vi "PID FRC form.vi"(4 "reinitialize? (F)":bool, 5 "output range":cluster{"output high":dbl, "output low":dbl}={"output high"=1.0, "output low"=-1.0} {"output low" format="%.2f"; "output high" format="%.2f"}, 6 "dt (s)":dbl=-1.0 format="%.3f", 7 "setpoint":dbl format="%.2f", 8 "d smoothing":dbl=nan format="%.2f", 9 "Feed Forward":dbl=1.5000000000000002, 10 "process variable":dbl format="%.2f", 11 "PID gains":T1={"proportional (Kc)"=1.0, "integral (Ki)"=0.01, "derivative (Kd)"=0.0} {"derivative (Kd)" format="%.3f"; "integral (Ki)" format="%.3f"; "proportional (Kc)" format="%.3f"}) -> (0 "dt out (s)":dbl format="%.3f", 1 "Chart":cluster{dbl, dbl}(graph), 3 "output":dbl format="%.2f")   [LabVIEW 2020]
doc: "Implements a PID that better meets FRC needs. It is in parallel form (Kp, Ki, Kd) and includes an arbitrary feedforward that is added to the output.\nThe PID algorithm features control output range limiting with integrator anti-windup and bumpless controller output for PID gain changes. The d smoothing (0-1) can help avoid oscillations caused by a stronger d term."
uses:
  <vilib>/addons/control/pid/pid.llb/PID Structure.ctl
  <vilib>/addons/control/pid/pid.llb/PID Structure Conversion (DBL).vi
  <vilib>/addons/control/pid/pid.llb/PID Advanced (DBL).vi
  <vilib>/addons/control/pid/NI_PID_pid.lvlib
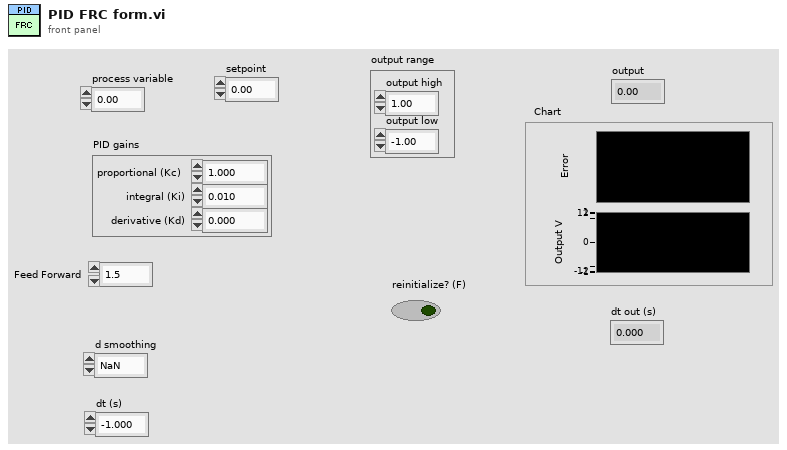
[diagram p1: front panel]
types:
  T1 = cluster{"proportional (Kc)":dbl, "integral (Ki)":dbl, "derivative (Kd)":dbl}
  T2 = typedef "NI_PID_pid.lvlib/PID Structure.ctl" = u16
  T3 = cluster{"proportional gain (Kc)":dbl, "integral time (Ti, min)":dbl, "derivative time (Td, min)":dbl}
  T4 = cluster{"proportional gain (Kc)":bool, "integral time (Ti, min)":bool, "derivative time (Td, min)":bool}
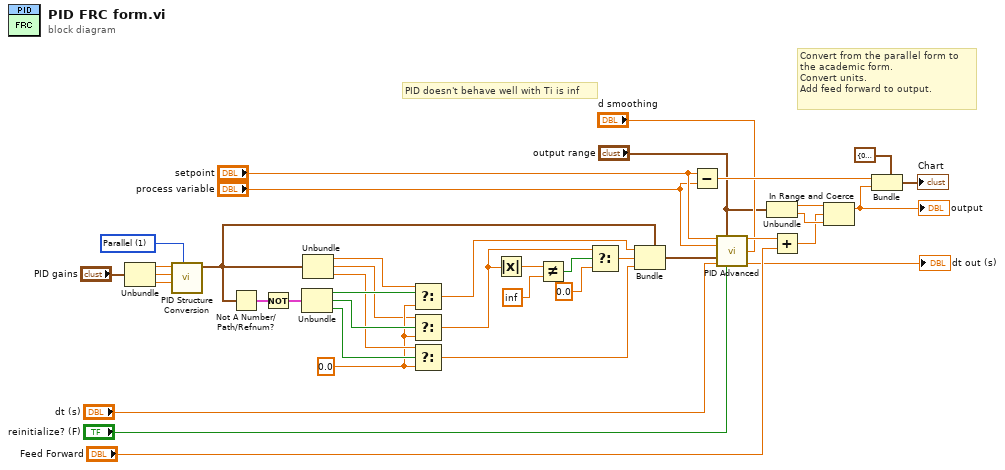
[diagram p0: block diagram]
diagram:
  w23 = 0.0
  w40 = T2 1 items=["Academic (Standard)", "Parallel", "Series"] ("PID structure")
  # "PID doesn't behave well with Ti is inf"
  # "Convert from the parallel form to\nthe academic form.\nConvert units.\nAdd feed forward to output."
  n1 = Unbundle("PID gains") -> ("proportional (Kc)"=w38:dbl, "integral (Ki)"=w37:dbl, "derivative (Kd)"=w36:dbl)
  n2 = call-poly <vilib>:"PID Structure Conversion.vi"("PID structure"=w40, "derivative"=w36, "integral"=w37, "proportional"=w38) -> ("PID gains"=w31:T3)  [unwired: 7 in]
  n3 = Not A Number/Path/Refnum?(number/path/refnum=w31) -> (NaN/Path/Refnum?=w30:T4)
  n4 = Not(x=w30) -> (.not. x?=w28:T4)
  n5 = Unbundle(w28) -> ("proportional gain (Kc)"=w29:bool, "integral time (Ti, min)"=w26:bool, "derivative time (Td, min)"=w25:bool)
  n6 = Unbundle(w31) -> ("proportional gain (Kc)"=w27:dbl, "integral time (Ti, min)"=w22:dbl, "derivative time (Td, min)"=w24:dbl)
  n7 = Select(t=w27, s=w29, f=w23) -> (s? t:f=w21:dbl)
  n8 = Select(t=w22, s=w26, f=w23) -> (s? t:f=w19:dbl)
  n9 = Select(t=w24, s=w25, f=w23) -> (s? t:f=w20:dbl)
  n10 = Absolute Value(x=w19) -> (abs(x)=w34:dbl)
  n11 = Not Equal?(x=w34, y=inf) -> (x != y?=w33:bool)
  n12 = Select(t=w19, s=w33, f=0.0) -> (s? t:f=w9:dbl)
  n13 = Bundle(cluster=w31, "proportional gain (Kc)"=w21, "integral time (Ti, min)"=w9, "derivative time (Td, min)"=w20) -> (w14:T3)
  n14 = Subtract(x="setpoint", y="process variable") -> (x-y=w12:dbl)
  n15 = call-poly <vilib>:"PID Advanced.vi"("setpoint"="setpoint", "output range"="output range", "process variable"="process variable", "alpha"="d smoothing", "PID gains"=w14, "dt (s)"="dt (s)", "reinitialize? (F)"="reinitialize? (F)") -> ("output"=w11:dbl, "dt out (s)"=→"dt out (s)":dbl)  [unwired: 7 in]
  n16 = Unbundle("output range") -> ("output high"=w5:dbl, "output low"=w4:dbl)
  n17 = Add(x=w11, y="Feed Forward") -> (x+y=w3:dbl)
  n18 = In Range and Coerce(upper limit=w5, x=w3, lower limit=w4) -> (coerced(x)=w2:dbl)  [unwired: 1 out]
  "output" <- w2
  n19 = Bundle(cluster=cluster{"Error":dbl, "output":dbl} {"Error"=0.0, "output"=0.0}, "Error"=w12, "output"=w2) -> (→"Chart":cluster{"Error":dbl, "output":dbl})
